vi "RVC Translation and Orientation.vi"() -> ()   [LabVIEW 2013]
uses:
  <vilib>/Analysis/baseanly.llb/Real A x B.vi
  <vilib>/Analysis/_algsub.llb/Vector Norm.vi
  <vilib>/Analysis/_algsub.llb/Real Vector Norm.vi
  <vilib>/Analysis/baseanly.llb/Outer Product.vi
  <vilib>/Analysis/baseanly.llb/Real Outer Product.vi
  <vilib>/robotics/Kinematics/Create Lie Group Matrix.vi
  <vilib>/Analysis/7linalg.llb/Create Special Matrix.vi
  <vilib>/Analysis/7linalg.llb/Create Special Real Matrix.vi
  <vilib>/Analysis/Matrix/Numeric/Multiply/Multiply.vi
  <vilib>/Analysis/Matrix/Numeric/Multiply/Multiply - RM,R.vi
  <vilib>/Analysis/Matrix/Numeric/Multiply/Multiply - R,RM.vi
  <vilib>/Analysis/Matrix/Numeric/Add/Add.vi
  <vilib>/Analysis/Matrix/Numeric/Add/Add - RM,RM.vi
  <vilib>/robotics/Kinematics/NI_Kinematics.lvlib
  <vilib>/Analysis/NI_AALBase.lvlib
panel:
  out "translation vector":dbl[](array[numeric]) format="%#.3f"
  out "rotation matrix":picture
  out "transformation matrix":picture
  in  "Position":dbl[](array[numeric])=[1.0, 1.0, 1.0]
  out "3D Picture":refnum<vi>(3d-picture)
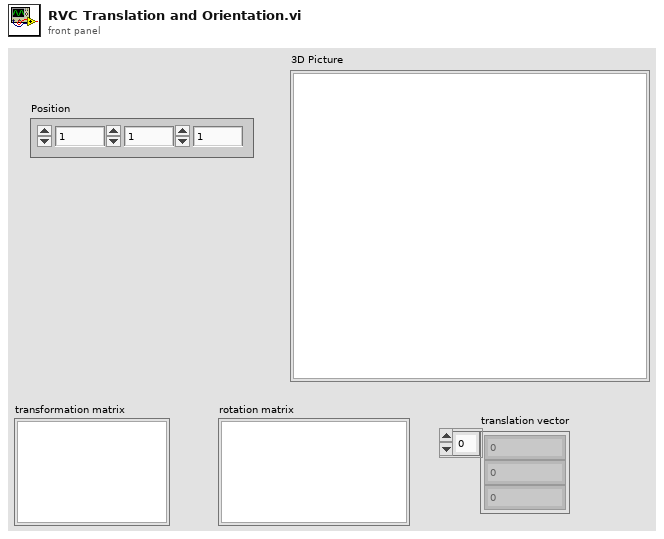
[diagram p1: front panel]
types:
  T1 = typedef "NI_Matrix.lvlib/RealMatrix.ctl" = dbl[][]
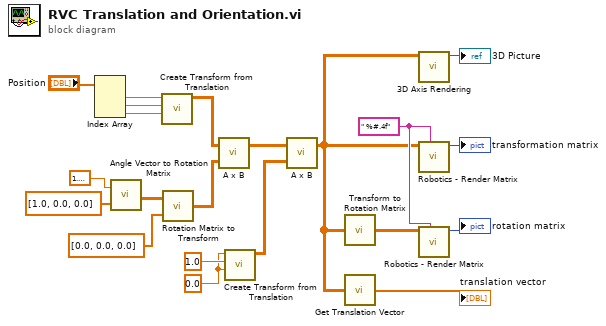
[diagram p0: block diagram]
diagram:
  w3 = " %#.4f" ("format string")
  w9 = 0.0 ("x")
  n1 = Index Array(array="Position") -> (element #1=w18:dbl, element #2=w17:dbl, element #3=w16:dbl)  [unwired: 3 in]
  n2 = call <vilib>:"Angle Vector to Rotation Matrix.vi"("vector"=dbl[] [1.0, 0.0, 0.0], "angle"=1.5707963267948966) -> ("rotation matrix"=w8:T1)
  n3 = call <vilib>:"Create Transform from Translation.vi"("z"=w16, "y"=w17, "x"=w18) -> ("transform"=w13:T1)  [unwired: 8 in]
  n4 = call <vilib>:"Rotation Matrix to Transform.vi"("translation vector"=dbl[] [0.0, 0.0, 0.0], "rotation matrix"=w8) -> ("transform"=w6:T1)
  n5 = call-poly <vilib>:"A x B.vi"("B"=w6, "A"=w13) -> ("A x B"=w10:T1)  [unwired: 1 out]
  n6 = call <vilib>:"Create Transform from Translation.vi"("z"=w9, "y"=1.0, "x"=w9) -> ("transform"=w11:T1)  [unwired: 8 in]
  n7 = call-poly <vilib>:"A x B.vi"("B"=w11, "A"=w10) -> ("A x B"=w2:T1)  [unwired: 1 out]
  n8 = call <vilib>:"Transform to Rotation Matrix.vi"("transform"=w2) -> ("rotation matrix"=w4:T1)
  n9 = call <vilib>:"Get Translation Vector.vi"("transform"=w2) -> ("translation vector"=→"translation vector":dbl[])
  n10 = call "3D Axis Rendering.vi"("rotation matrix"=w2) -> ("SceneNode out"=→"3D Picture":refnum<vi>)  [unwired: 10 in]
  n11 = call "Robotics - Render Matrix.vi"("format string"=w3, "A"=w2) -> ("picture out"=→"transformation matrix":picture)  [unwired: 9 in]
  n12 = call "Robotics - Render Matrix.vi"("format string"=w3, "A"=w4) -> ("picture out"=→"rotation matrix":picture)  [unwired: 9 in]
